vi "Write Creation TS.vi"(8 "error in (no error)":errorcluster, 10 "Start Creation":u64, 11 "CIFCorePlugin in":refnum<class "CIFCorePlugin.lvclass">) -> (0 "error out":errorcluster, 3 "CIFCorePlugin out":refnum<class "CIFCorePlugin.lvclass">)   [LabVIEW 2021, in "CIFCorePlugin.lvclass"]
doc: "Update the timestamp. Time is U64, absolute time in nS in the appropriate clockID configured for the plugin. If a 0 is wired it will automatically get the current time."
uses:
  CIFCorePlugin.lvclass
  CIFCorePlugin.lvclass/CIFCorePlugin.ctl
  Get Time.vi
  CIFUtilities/CIFClocks/Core/Get Time.vi
  CIFUtilities/CIFClocks/Time Conversion/LabVIEW Time to UTC Time.vi
  Common/Utilities/Add Error.vi
  Common/Utilities/Append Error Location.vi
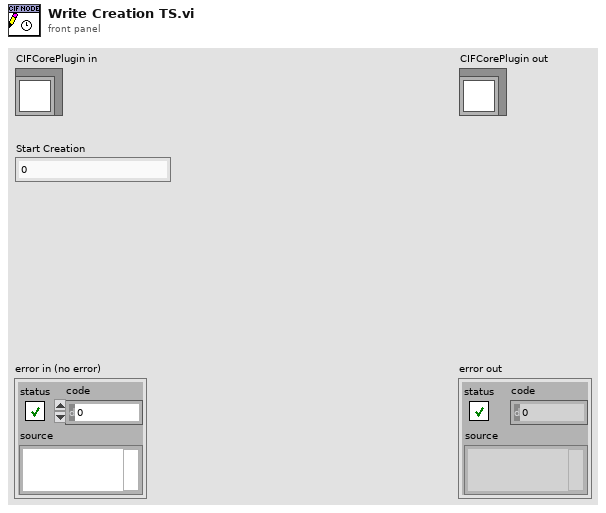
[diagram p1: front panel]
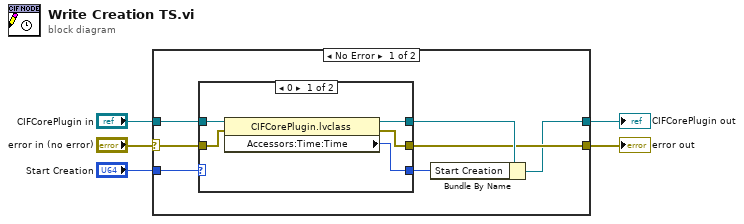
[diagram p0: block diagram]
diagram:
  n1 = case shown="No Error" "error in (no error)" {
    selector: "error in (no error)" -> [w11 w21]
    tunnel: [w7 w21] -> w4
    tunnel: [w6 w22] -> w2
    tunnel: "CIFCorePlugin in" -> [w10 w22]
    tunnel: "Start Creation" -> [w12 _]
    frame No Error {
      n2 = case shown="0" w12 {
        selector: w12 -> [_ w19]
        tunnel: w11 -> [w14 w18]
        tunnel: w10 -> [w17 w20]
        tunnel: [w16 w20] -> w9
        tunnel: [w15 w19] -> w8
        tunnel: [w13 w18] -> w7
        frame 0 {
          n3 = property class="CIFCorePlugin.lvclass"(reference=w17, error in=w14) -> (reference out=w16:refnum<class "CIFCorePlugin.lvclass">, error out=w13:errorcluster, "Accessors:Time:Time"=w15:u64)
        }
        frame 1, Default {
        }
      }
      n4 = Bundle By Name(cluster=w9, "Start Creation"=w8) -> (w6:refnum<class "CIFCorePlugin.lvclass">)
    }
    frame Error {
    }
  }
  "error out" <- w4
  "CIFCorePlugin out" <- w2
